vi "Google Earth - View Extents.vi"(8 "error in":errorcluster, 11 "Refnum In":refnum<k7>) -> (0 "error out":errorcluster, 2 "Extents":T1, 3 "Refnum Out":refnum<k7>)   [LabVIEW 2009]
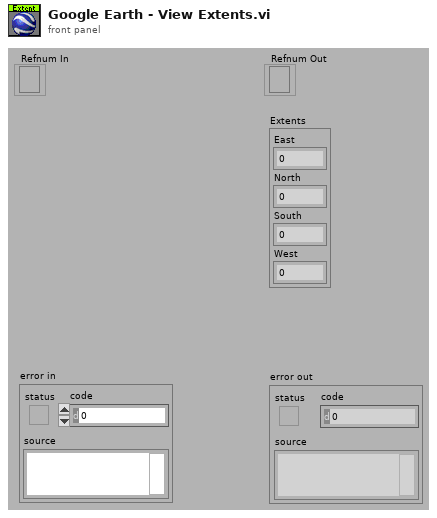
[diagram p1: front panel]
types:
  T1 = cluster{"East":dbl, "North":dbl, "South":dbl, "West":dbl}
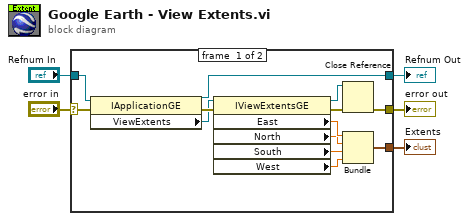
[diagram p0: block diagram]
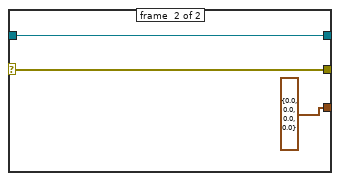
[diagram p2: hidden frame]
diagram:
  n1 = case shown="No Error" "error in" {
    selector: "error in" -> [w6 w21]
    tunnel: [w18 T1 {"East"=0.0, "North"=0.0, "South"=0.0, "West"=0.0}] -> w5
    tunnel: [w13 w20] -> w4
    tunnel: "Refnum In" -> [w12 w20]
    tunnel: [w7 w21] -> w2
    frame #0 {
      n2 = property class="IApplicationGE"(reference=w12, error in=w6) -> (reference out=w13:refnum<k7>, error out=w9:errorcluster, "ViewExtents"=w8:refnum<k7>)
      n3 = property class="IViewExtentsGE"(reference=w8, error in=w9) -> (reference out=w11:refnum<k7>, error out=w10:errorcluster, "East"=w16:dbl, "North"=w15:dbl, "South"=w14:dbl, "West"=w17:dbl)
      n4 = Close Reference(reference=w11, error in (no error)=w10) -> (error out=w7:errorcluster)
      n5 = Bundle("East"=w16, "North"=w15, "South"=w14, "West"=w17) -> (w18:T1)  [unwired: 1 in]
    }
    frame #1 {
    }
  }
  "Extents" <- w5
  "Refnum Out" <- w4
  "error out" <- w2
